vi "Read PUBREC.vi"(8 "error in (no error)":errorcluster, 11 "connection ID":refnum<k5>) -> (0 "error out":errorcluster, 2 "Message ID":u16=10 format="%x", 3 "connection ID out":refnum<k5>)   [LabVIEW 2020, in "DAQIO MQTT.lvlib"]
doc: "© 2015 - daq.io, LLC - Peter Adelhardt"
uses:
  DAQIO MQTT.lvlib
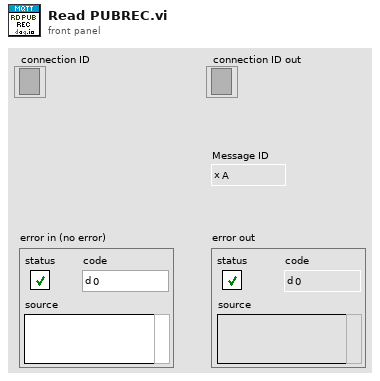
[diagram p1: front panel]
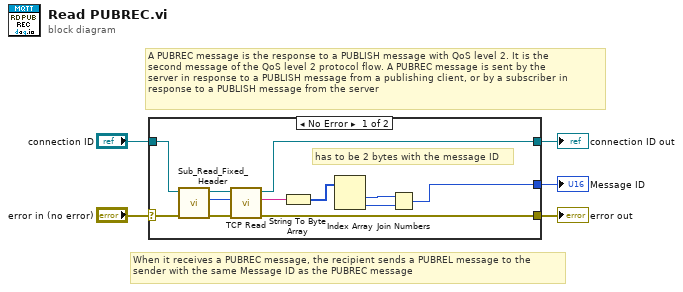
[diagram p0: block diagram]
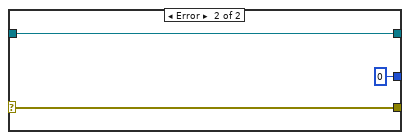
[diagram p2: hidden frame]
diagram:
  # "When it receives a PUBREC message, the recipient sends a PUBREL message to the\nsender with the same Message ID as the PUBREC message"
  # "A PUBREC message is the response to a PUBLISH message with QoS level 2. It is the\nsecond message of the QoS level 2 protocol flow. A PUBREC message is sent by the\nserver in response to a PUBLISH message from a publishing client, or by a subscriber in\nresponse to a PUBLISH message from the server"
  n1 = case shown="No Error" "error in (no error)" {
    selector: "error in (no error)" -> [w16 w20]
    tunnel: [w10 w20] -> w4
    tunnel: "connection ID" -> [w8 w18]
    tunnel: [w7 w18] -> w2
    tunnel: [w6 u16 0] -> w1
    frame No Error {
      # "has to be 2 bytes with the message ID"
      n2 = call "Sub_Read_Fixed_Header.vi"("error in (no error)"=w16, "connection ID"=w8) -> ("error out"=w11:errorcluster, "Remaining Length"=w17:u32, "connection ID out"=w9:refnum<k5>)  [unwired: 3 in, 4 out]
      n3 = call "TCP Read.vi"("error in (no error)"=w11, "bytes to read"=w17, "connection ID"=w9) -> ("error out"=w10:errorcluster, "data out"=w12:string, "connection ID out"=w7:refnum<k5>)  [unwired: 6 in]
      n4 = String To Byte Array(string=w12) -> (unsigned byte array=w13:u8[])
      n5 = Index Array(array=w13) -> (element #1=w15:u8, element #2=w14:u8)  [unwired: 2 in]
      n6 = Join Numbers(hi=w15, lo=w14) -> ((hi.lo)=w6:u16)
    }
    frame Error {
    }
  }
  "error out" <- w4
  "Message ID" <- w1
  "connection ID out" <- w2
